vi "SetSubRegion.vi"(8 "error in (no error)":errorcluster, 10 "ROI":T3, 11 "HAMAMATSU_DCAMAPI in":refnum<class "HAMAMATSU_DCAMAPI.lvclass">) -> (0 "error out":errorcluster, 3 "HAMAMATSU_DCAMAPI out":refnum<class "HAMAMATSU_DCAMAPI.lvclass">)   [LabVIEW 2020, in "HAMAMATSU_DCAMAPI.lvclass"]
uses:
  HAMAMATSU_DCAMAPI.lvclass
  <vilib>/Utility/miscctls.llb/LVMinMaxIncTypeDef.ctl
  HAMAMATSU_DCAMAPI.lvclass/HAMAMATSU_DCAMAPI.ctl
panel:
  out "Sub Region":T2 {"V Size"."Value" min=0 max=0 step=4; "H Size"."Value" min=0 max=0 step=4; "V Offset"."Value" min=0 max=0 step=4; "H Offset"."Value" min=0 max=0 step=4}
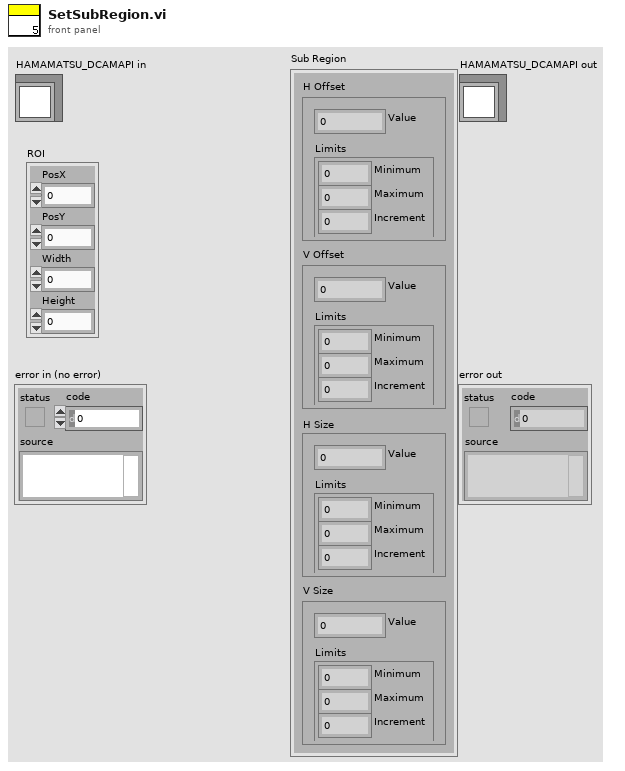
[diagram p1: front panel]
types:
  T1 = typedef "LVMinMaxIncTypeDef.ctl" = cluster{"Minimum":dbl, "Maximum":dbl, "Increment":dbl}
  T2 = cluster{"H Offset":cluster{"Value":i32, "Limits":T1}, "V Offset":cluster{"Value":i32, "Limits":T1}, "H Size":cluster{"Value":i32, "Limits":T1}, "V Size":cluster{"Value":i32, "Limits":T1}}
  T3 = cluster{"PosX":i32, "PosY":i32, "Width":i32, "Height":i32}
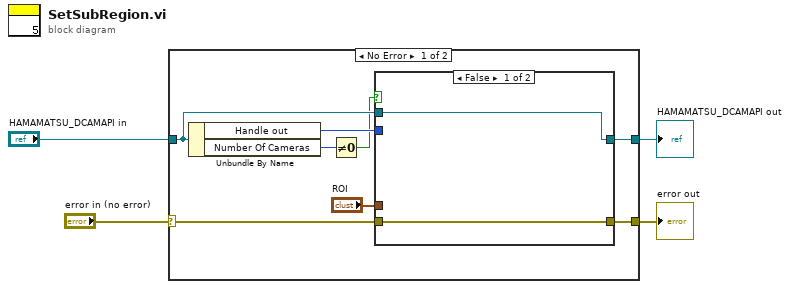
[diagram p0: block diagram]
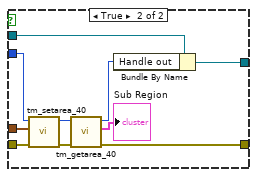
[diagram p2: hidden frame]
diagram:
  n1 = case shown="No Error" "error in (no error)" {
    selector: "error in (no error)" -> [w9 w25]
    tunnel: [w12 w25] -> w4
    tunnel: "HAMAMATSU_DCAMAPI in" -> [w8 w26]
    tunnel: [w10 w26] -> w2
    frame No Error {
      n2 = Unbundle By Name(w8) -> ("Handle out"=w7:u32, "Number Of Cameras"=w6:u32)
      n3 = Not Equal To 0?(x=w6) -> (x != 0?=w5:bool)
      n4 = case shown="False" w5 {
        tunnel: w9 -> [w13 w22]
        tunnel: [w13 w21] -> w12
        tunnel: "ROI" -> [_ w20]
        tunnel: w8 -> [w14 w19]
        tunnel: [w14 w18] -> w10
        tunnel: w7 -> [_ w16]
        frame False {
        }
        frame True {
          n5 = call <userlib>:"tm_setarea_40.vi"("error in (no error)"=w22, "Sub Region"=w20, "Handle in"=w16) -> ("error out"=w23:errorcluster, "Handle out"=w24:u32)  [unwired: 7 in]
          n6 = call <userlib>:"tm_getarea_40.vi"("error in (no error)"=w23, "Handle in"=w24) -> ("error out"=w21:errorcluster, "Sub Region"=→"Sub Region":T2, "Handle out"=w17:u32)  [unwired: 7 in]
          n7 = Bundle By Name(cluster=w19, "Handle out"=w17) -> (w18:refnum<class "HAMAMATSU_DCAMAPI.lvclass">)
        }
      }
    }
    frame Error {
    }
  }
  "error out" <- w4
  "HAMAMATSU_DCAMAPI out" <- w2
